vi "Handle Error.vi"(8 "error in (no error)":errorcluster, 11 "MVVM Abstruct Controller in":refnum<class "MVVM Abstruct Controller.lvclass">) -> (0 "error out":errorcluster, 2 "stop actor?":bool=TRUE, 3 "MVVM Abstruct Controller out":refnum<class "MVVM Abstruct Controller.lvclass">)   [LabVIEW 2020, in "MMVVM Framework.lvlib" / "MVVM Abstruct Controller.lvlib" / "MVVM Abstruct Controller.lvclass"]
doc: "(<B>Filename</B>: Actor Framework.lvlib:Actor.lvclass:Handle Error.vi)\n\nDefines how the actor handles an error that occurred while processing a message. By default, this method does nothing except stop the actor."
uses:
  MVVM Abstruct Controller.lvclass
  Abstruct View/Abstruct View/Abstruct View.lvclass
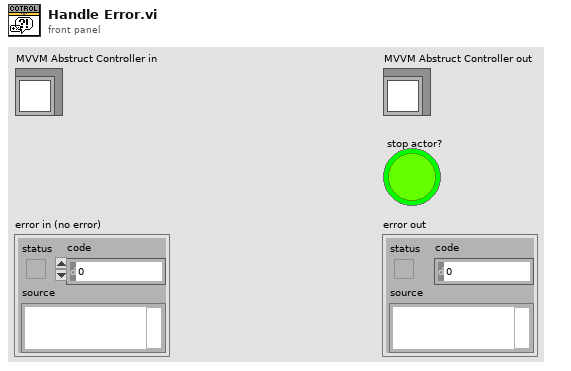
[diagram p1: front panel]
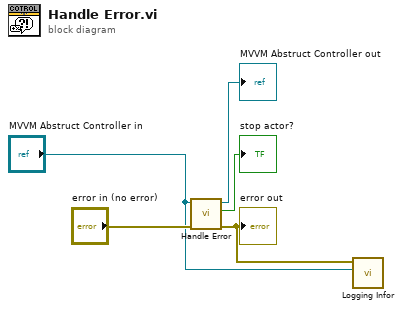
[diagram p0: block diagram]
diagram:
  n1 = call-parent "Handle Error.vi"("error in (no error)"="error in (no error)", "Actor in"="MVVM Abstruct Controller in") -> ("error out"=w2:errorcluster, "stop actor?"=→"stop actor?":bool, "Actor out"=→"MVVM Abstruct Controller out":refnum<class "MVVM Abstruct Controller.lvclass">)  [unwired: 7 in]
  "error out" <- w2
  n2 = call "Logging Infor.vi"("Class"="MVVM Abstruct Controller in", "error in (no error)"=w2) -> ()  [unwired: 9 in, 1 out]
